vi "Vision Research Phantom Series Register Client.vi"(0 "Storage Path (\"\")":path=path "C:/ProgramData/Phantom/787", 5 "Error In (no error)":errorcluster, 7 "CallID":u32) -> (14 "HRESULT":i32, 19 "Error Out":errorcluster)   [LabVIEW 2013, in "VRI.lvlib"]
doc: "PhCon.dll\n\nPhLVRegisterClientEx\nHRESULT PhLVRegisterClientEx(char *szStgPath, UINT CallID, UINT PhConHeaderVersion)\n\nParameters Description\nszStgPath (in) The path for the stg files for the cameras. It may be your\n exe path or your StartIn path.\nCallID (in) User CallID for progress indicator\nPhConHeaderVersion (in) PhCon library version. You must pass the value of \n PHCONHEADERVERSION symbol defined in PhCon.h\nReturn HRESULT (0=Ok)\nComments This function registers an application as a client of this dll\n and provides the path for the serial tag files of the cameras.\n\nWritten by:\nBLOOMY CONTROLS, INC\nWINDSOR, CT 06095, USA\n860-298-9925\nwww.bloomy.com\nV1.0.0\nMay, 2004"
uses:
  VRI.lvlib
  Phantom DLLs/PhCon.Dll
panel:
  # "For instructions on the use of this VI, press Ctrl+H to display the help window and move the mouse over the icon, controls, and indicators"
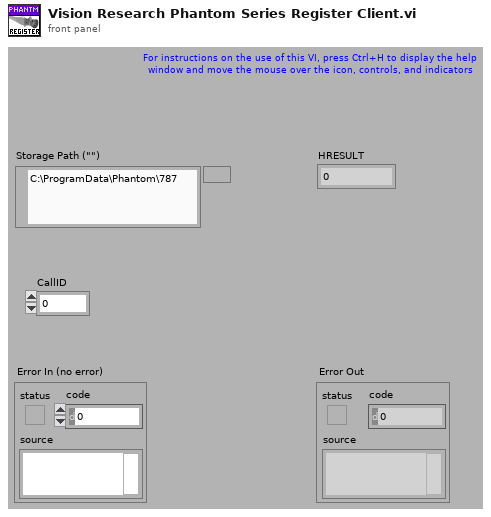
[diagram p1: front panel]
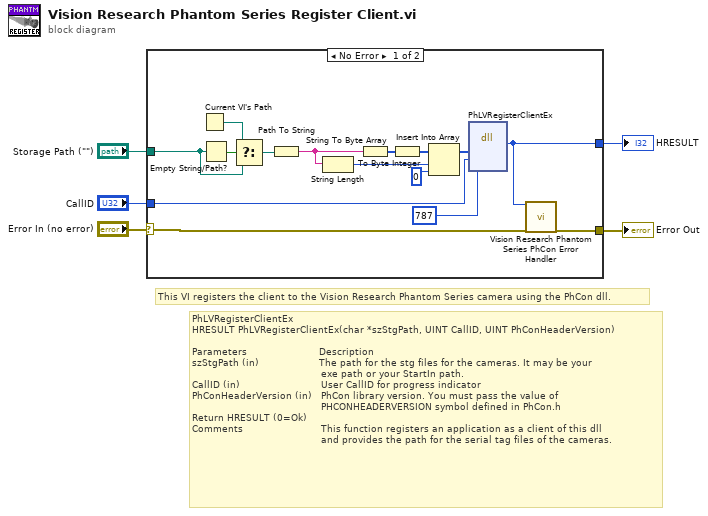
[diagram p0: block diagram]
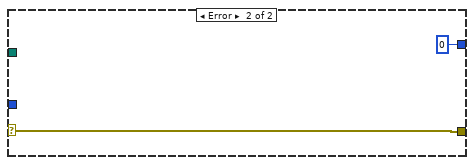
[diagram p2: hidden frame]
diagram:
  # "PhLVRegisterClientEx\nHRESULT PhLVRegisterClientEx(char *szStgPath, UINT CallID, UINT PhConHeaderVersion)\n\nParameters                        Description\nszStgPath (in)                    The path for the stg files for the cameras. It may be your\n                                           exe path or your StartIn path.\nCallID (in)                           User CallID for progress indicator\nPhConHeaderVersion (in)   PhCon library version. You must pass the value of \n                                           PHCONHEADERVERSION symbol defined in PhCon.h\nReturn HRESULT (0=Ok)\nComments                          This function registers an application as a client of this dll\n                                           and provides the path for the serial tag files of the cameras."
  # "This VI registers the client to the Vision Research Phantom Series camera using the PhCon dll."
  n1 = case shown="No Error" "Error In (no error)" {
    selector: "Error In (no error)" -> [w20 w22]
    tunnel: [w19 w22] -> w4
    tunnel: "Storage Path (\"\")" -> [w18 _]
    tunnel: [w17 0] -> w2
    tunnel: "CallID" -> [w16 _]
    frame No Error {
      n2 = Current VI's Path() -> (path=w8:path)
      n3 = Empty String/Path?(string/path=w18) -> (empty?=w9:bool)
      n4 = Select(t=w8, s=w9, f=w18) -> (s? t:f=w7:path)
      n5 = Path To String(path=w7) -> (string=w10:string)
      n6 = String Length(string=w10) -> (length=w15:i32)
      n7 = String To Byte Array(string=w10) -> (unsigned byte array=w14:u8[])
      n8 = To Byte Integer(number=w14) -> (8bit integer=w11:i8[])
      n9 = Insert Into Array(array=w11, index=w15, new element=i8 0) -> (w12:i8[])
      n10 = dll-call lib="C:/Projects/SDK/64-bit/Vision Research Phantom Series Labview Driver/Phantom DLLs/PhCon.dll" fn="PhLVRegisterClientEx"("pStgPath"=w12, "CallID"=w16, "PhConHeaderVersion"=787) -> ("return type"=w17:i32)  [unwired: 6 in, 2 out]
      n11 = call "Vision Research Phantom Series PhCon Error Handler.vi"("ErrNo"=w17, "Error In (no error)"=w20) -> ("Error Out"=w19:errorcluster)  [unwired: 17 out]
    }
    frame Error {
    }
  }
  "Error Out" <- w4
  "HRESULT" <- w2
